vi "_Load XML Method.vi"(8 "Path":path=path "C:/Users/Min/Documents/Software Design/Requests/Method Tunner/Mode Switching-ESI1-APCI2-Molana.xml") -> (0 "error out":errorcluster, 1 "ExptParamAndMR":T2(array[cluster]), 2 "Experiment List":string[][](array[string]), 3 "MethodLevelParameters":string[][](array[string]), 4 "DOM document":refnum<k20>)   [LabVIEW 2012]
uses:
  Type/_Mass Range Parameters.ctl
  <vilib>/xml/Load XML File.vi
  <vilib>/xml/Close Reference(Node).vi
  <vilib>/xml/NI_XML.lvlib
  <resource>/objmgr/DOMUserDefRef.rc
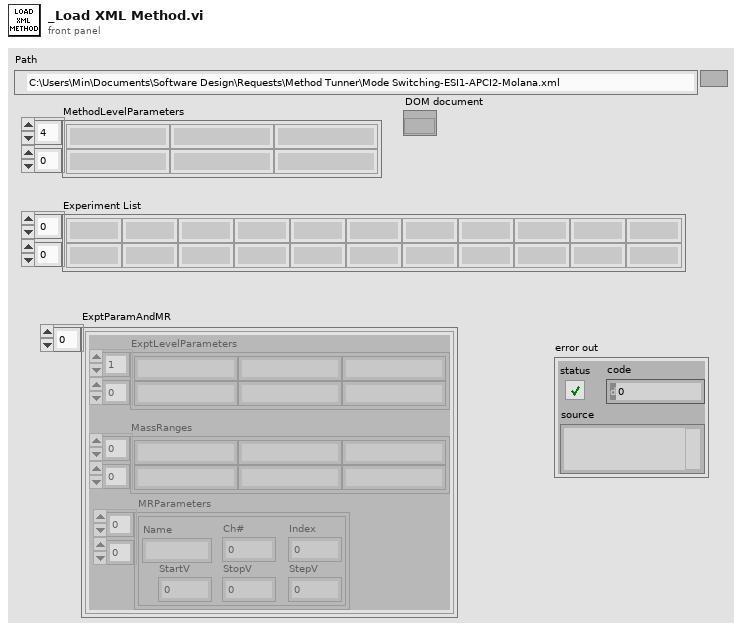
[diagram p1: front panel]
types:
  T1 = typedef "_Mass Range Parameters.ctl" = cluster{"Name":string, "Ch#":u8, "StartV":dbl, "StopV":dbl, "StepV":dbl, "Index":u8}
  T2 = cluster{"ExptLevelParameters":string[][], "MassRanges":string[][], " MRParameters":T1[][]}[]
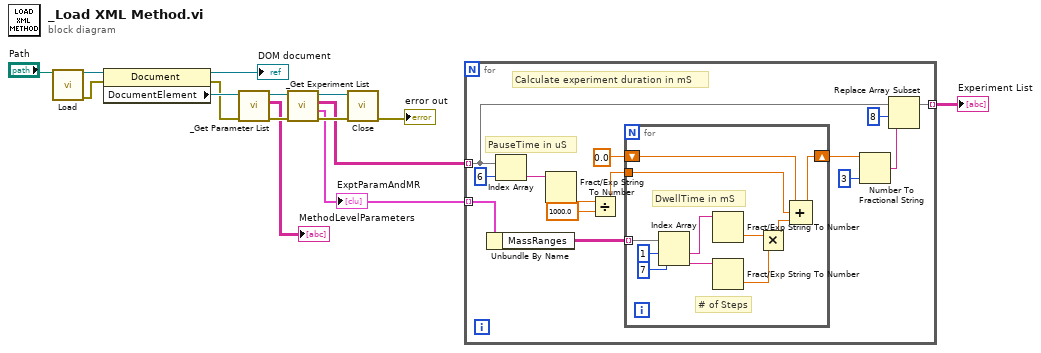
[diagram p0: block diagram]
diagram:
  n1 = call-poly <vilib>:"Load.vi"("path to XML document"="Path") -> ("DOM document out"=w15:refnum<k20>, "error out"=w14:errorcluster)  [unwired: 12 in, 1 out]
  n2 = property on="Property Node" class="Document"(reference=w15, error in=w14) -> (reference out=→"DOM document":refnum<k20>, error out=w7:errorcluster, "DocumentElement"=w10:refnum<k20>)
  n3 = call "_Get Parameter List.vi"("error in (no error)"=w7, "node in"=w10) -> ("error out"=w8:errorcluster, "Parameters List"=→"MethodLevelParameters":string[][], "node out"=w9:refnum<k20>)  [unwired: 3 in]
  n4 = call "_Get Experiment List.vi"("error in (no error)"=w8, "node in"=w9) -> ("error out"=w11:errorcluster, "ExptParamAndMR"=w3:T2, "Expt"=w2:string[][], "node out"=w13:refnum<k20>)  [unwired: 2 in]
  "ExptParamAndMR" <- w3
  n5 = call-poly <vilib>:"Close.vi"("error in (no error)"=w11, "node"=w13) -> ("error out"=→"error out":errorcluster)  [unwired: 7 in]
  n6 = for {
    tunnel: w2 -> [w19] mode=indexing
    tunnel: w3 -> [w25] mode=indexing
    tunnel: [w16] -> w1 mode=indexing
    # "PauseTime in uS"
    # "Calculate experiment duration in mS"
    n7 = Unbundle By Name(w25) -> ("MassRanges"=w24:string[][])
    n8 = Index Array(array=w19, index=6) -> (element=w28:string)
    n9 = Fract/Exp String To Number(string=w28) -> (number=w27:dbl)  [unwired: 3 in, 1 out]
    n10 = Divide(x=w27, y=1000.0) -> (x/y=w23:dbl)
    n11 = for {
      tunnel: w24 -> [w40] mode=indexing
      tunnel: w23 -> [w32]
      shift-right: [w30] -> w21
      shift-left: 0.0 -> [w31]
      # "# of Steps"
      # "DwellTime in mS"
      n12 = Index Array(array=w40, index #1=1 ("index"), index #2=7 ("index")) -> (element #1=w36:string, element #2=w37:string)
      n13 = Fract/Exp String To Number(string=w36) -> (number=w35:dbl)  [unwired: 3 in, 1 out]
      n14 = Fract/Exp String To Number(string=w37) -> (number=w34:dbl)  [unwired: 3 in, 1 out]
      n15 = Multiply(x=w35, y=w34) -> (x*y=w33:dbl)
      n16 = Compound Arithmetic op=ADD(w31, w32, w33) -> (w30:dbl)
    }
    n17 = Number To Fractional String(number=w21, precision (6)=i16 3) -> (F-format string=w17:string)  [unwired: 2 in]
    n18 = Replace Array Subset(array=w19, new element=w17, index=8) -> (w16:string[])
  }
  "Experiment List" <- w1
